vi "Read test seq.vi"(3 "In data":string[][](array[string])) -> (1 "Out Data":string[][](array[string]))   [LabVIEW 2017]
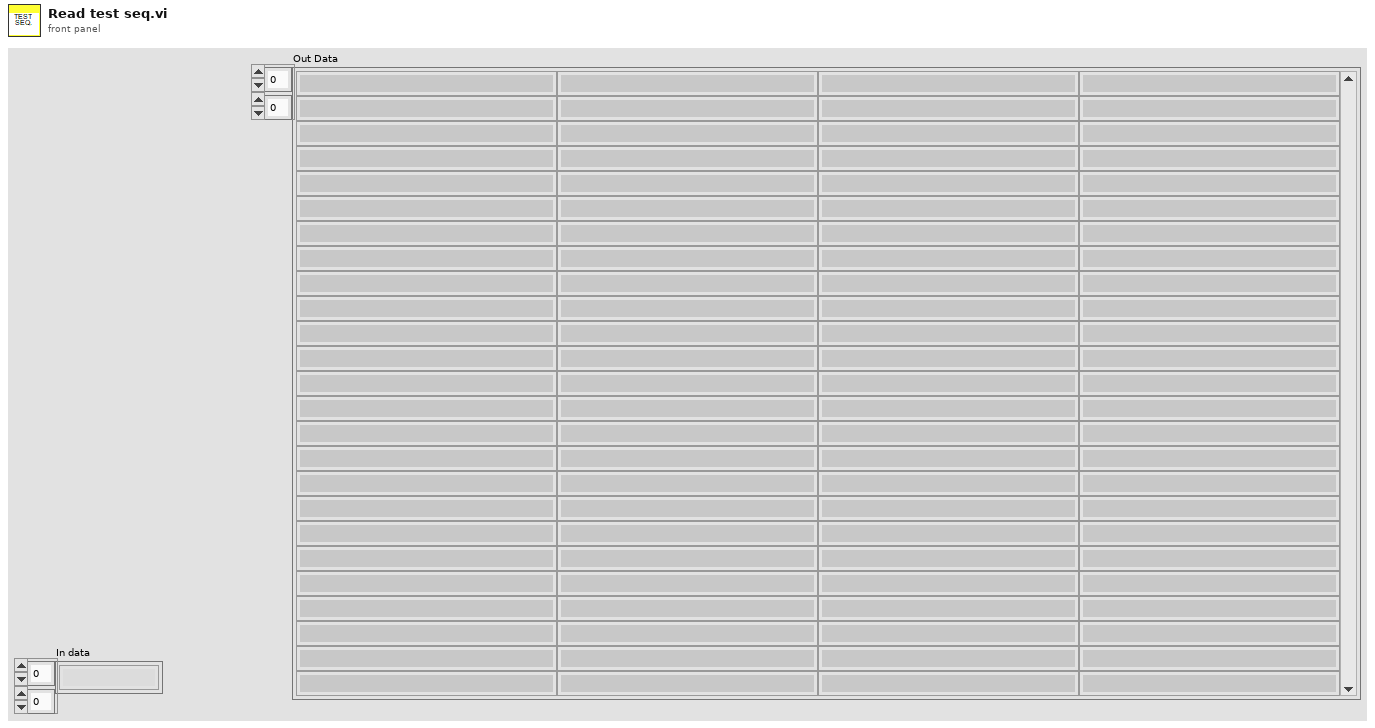
[diagram p1: front panel]
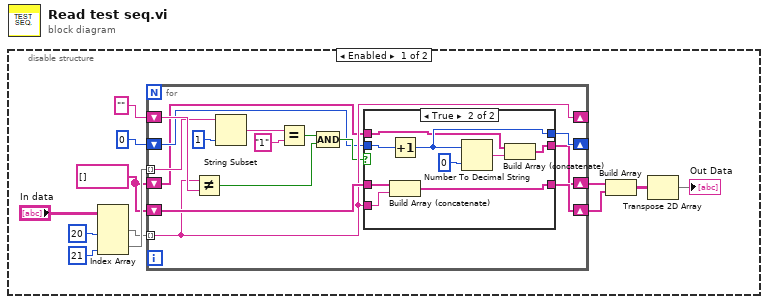
[diagram p0: block diagram]
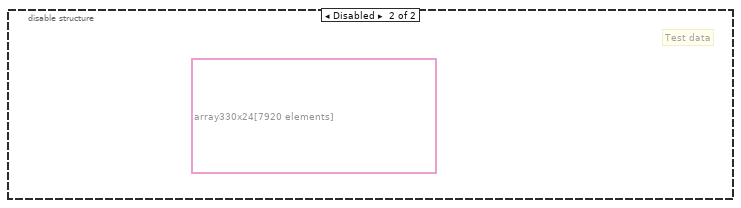
[diagram p3: hidden frame]
diagram:
  n1 = disable-structure shown="Enabled" {
    frame Enabled {
      w2 = string[] []
      n2 = Index Array(array="In data", index (col) #1=20 ("disabled index (col)"), index (col) #2=21 ("index (col)")) -> (element #1=w9:string[], element #2=w10:string[])  [unwired: 2 in]
      n3 = for {
        tunnel: w10 -> [w17] mode=indexing
        tunnel: w9 -> [w22] mode=indexing
        shift-right: [w24] -> w5
        shift-left: w2 -> [w26]
        shift-right: [w22] -> _
        shift-left: "" -> [w23]
        shift-right: [w15] -> _
        shift-left: 0 -> [w16]
        shift-right: [w14] -> w6
        shift-left: w2 -> [w13]
        n4 = Not Equal?(x=w22, y=w23) -> (x != y?=w20:bool)
        n5 = String Subset(string=w17, length (rest)=1 ("length (rest)")) -> (substring=w19:string)  [unwired: 1 in]
        n6 = Equal?(x=w19, y="1") -> (x = y?=w25:bool)
        n7 = Compound Arithmetic op=AND(w25, w20) -> (w21:bool)
        n8 = case shown="True" w21 {
          tunnel: w26 -> [w30 w34]
          tunnel: w22 -> [_ w35]
          tunnel: [w30 w33] -> w24
          tunnel: w16 -> [w29 w39]
          tunnel: [w29 w37] -> w15
          tunnel: [w28 w32] -> w14
          tunnel: w13 -> [w28 w31]
          frame False {
          }
          frame True {
            n9 = Increment(x=w39) -> (x+1=w37:i32)
            n10 = Build Array (concatenate)(w34, w35) -> (w33:string[])
            n11 = Number To Decimal String(number=w37, width (-)=i16 0) -> (decimal integer string=w36:string)
            n12 = Build Array (concatenate)(w31, w36) -> (w32:string[])
          }
        }
      }
      n13 = Build Array(w6, w5) -> (w4:string[][])
      n14 = Transpose 2D Array(2D array=w4) -> (transposed array=→"Out Data":string[][])
    }
    frame Disabled {
      (unwired) string[][] array330x24[7920 elements] ("Actual_SEQ")
      # "Test data"
    }
  }
